vi "CheckName.vi"(8 "error in (no error)":errorcluster, 11 "input array":string[](array[string])) -> (0 "error out":errorcluster, 3 "duplicated?":bool)   [LabVIEW 2009]
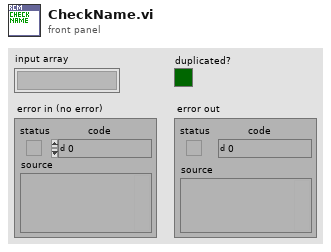
[diagram p1: front panel]
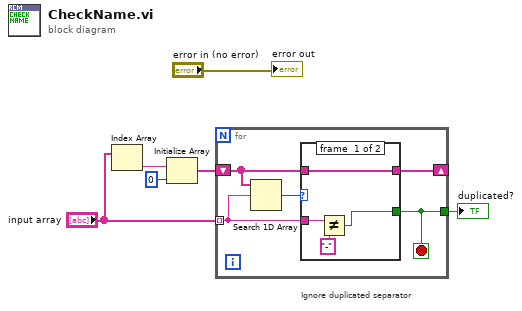
[diagram p0: block diagram]
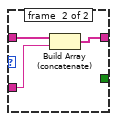
[diagram p2: hidden frame]
diagram:
  # "Ignore duplicated separator"
  n1 = Index Array(array="input array") -> (element=w6:string)  [unwired: 1 in]
  n2 = Initialize Array(w6, 0 ("dimension size")) -> (w4:string[])
  n3 = for {
    tunnel: "input array" -> [w8] mode=indexing
    shift-right: [w9] -> _
    shift-left: w4 -> [w10]
    tunnel: [w7] -> w2
    stop <- w7 stop-if-true
    n4 = Search 1D Array(1D array=w10, element=w8) -> (index of element=w11:i32)  [unwired: 1 out]
    n5 = case shown="0, Default" w11 {
      tunnel: w10 -> [w15 w18]
      tunnel: [w15 w17] -> w9
      tunnel: w8 -> [w14 w16]
      tunnel: [w12 _] -> w7
      frame #0 {
        n6 = Not Equal?(x=w14, y="-") -> (x != y?=w12:bool)
      }
      frame #1 {
        n7 = Build Array (concatenate)(w18, w16) -> (w17:string[])
      }
    }
  }
  "duplicated?" <- w2
  "error out" <- "error in (no error)"
